vi "Read Files from m-File.vi"(8 "error in":errorcluster, 11 "File Path":path) -> (0 "error out":errorcluster, 3 "Paths":path[](array[path]))   [LabVIEW 2020]
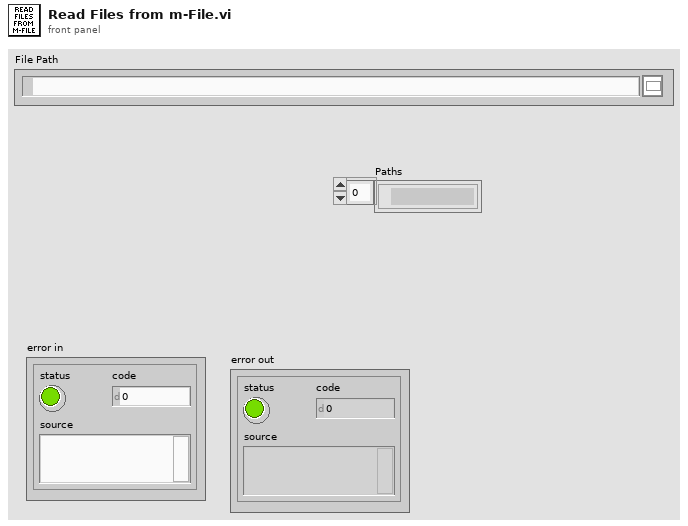
[diagram p1: front panel]
types:
  T1 = enum16{"open", "open or create", "create or replace", "create", "open (read-only)"}
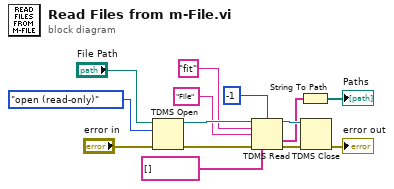
[diagram p0: block diagram]
diagram:
  n1 = TDMS Open(8:"error in", 10:T1."open (read-only)" ("operation (0:open)"), 11:"File Path") -> (0:w11:errorcluster, 3:w10:refnum<k34>)  [unwired: 4 in]
  n2 = TDMS Read(0:w10, 2:i64 -1 ("count (-1: all)"), 5:"fit" ("group name in"), 7:"File", 11:w11, 12:string[] []) -> (4:w6:refnum<k34>, 10:w2:string[], 15:w8:errorcluster)  [unwired: 2 in, 3 out]
  n3 = String To Path(string=w2) -> (path=→"Paths":path[])
  n4 = TDMS Close(8:w8, 11:w6) -> (0:→"error out":errorcluster)  [unwired: 1 out]
